vi "live data display.vi"(11 "queue":refnum<queue>) -> ()   [LabVIEW 2018]
uses:
  state.ctl
  liveData cluster.ctl
panel:
  out "STOP":bool
  out "Waveform Graph":dbl[](graph)
  in  "mode":bool
  in  "channel":u16(ring)
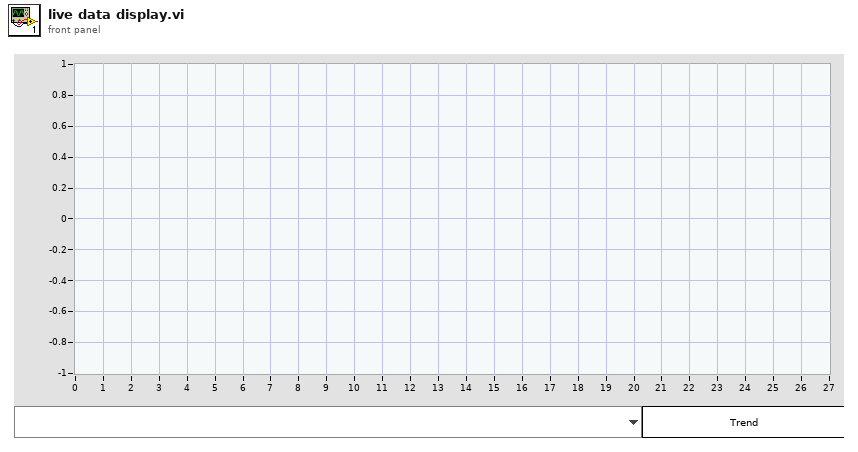
[diagram p1: front panel]
types:
  T1 = typedef "liveData cluster.ctl" = cluster{"channelSelection":i32, "length":dbl, "history":dbl[], "Trend":bool, "plotRef":refnum<vi>}
  T2 = typedef "state.ctl" = enum16{"readData", "init", "channel", "mode", "quit"}
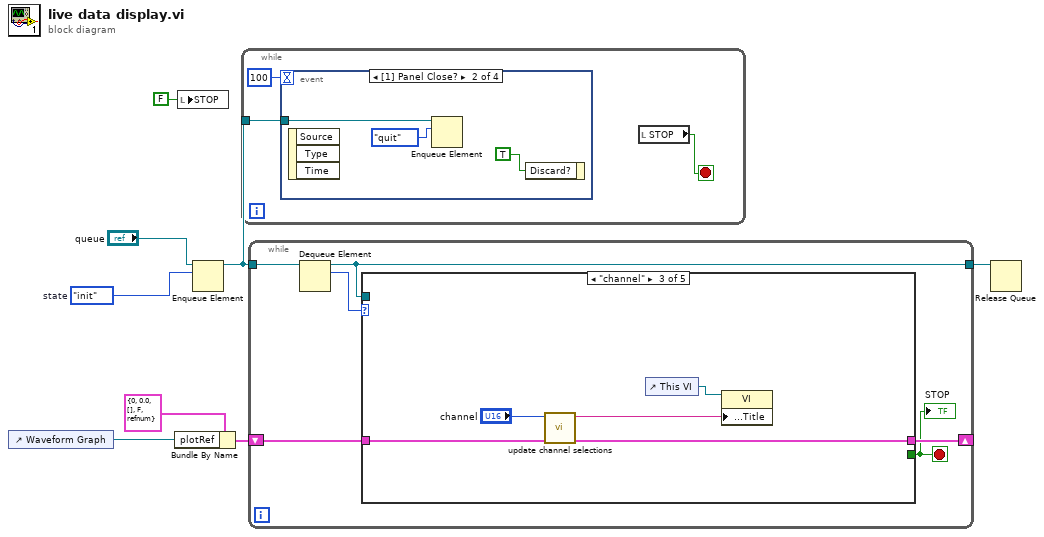
[diagram p0: block diagram]
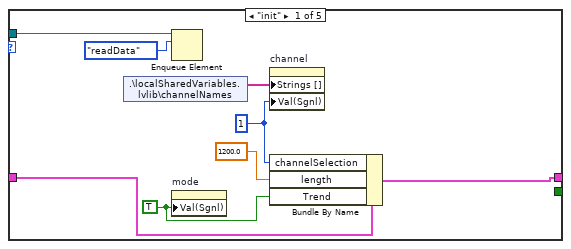
[diagram p2: hidden frame]
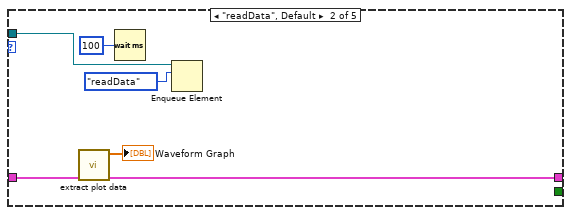
[diagram p3: hidden frame]
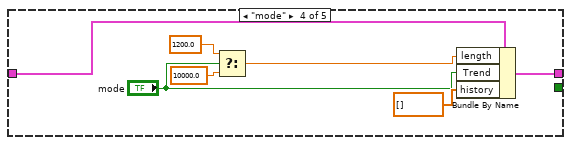
[diagram p4: hidden frame]
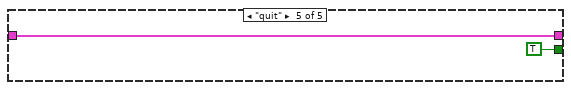
[diagram p5: hidden frame]
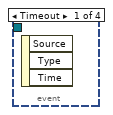
[diagram p6: hidden frame]
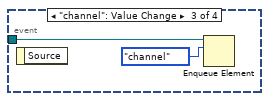
[diagram p7: hidden frame]
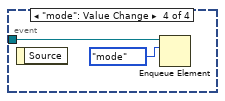
[diagram p8: hidden frame]
diagram:
  w3 = state."init"  # state
  n1 = control-ref of="Waveform Graph"() -> (w4:refnum<vi>)
  n2 = Bundle By Name(cluster=T1 {"channelSelection"=0, "length"=0.0, "history"=[], "Trend"=FALSE, "plotRef"=refnum}, "plotRef"=w4) -> (w5:T1)
  n3 = local write "STOP"(FALSE ("STOP")) -> ()
  n4 = Enqueue Element(queue="queue", element=w3) -> (queue out=w6:refnum<queue>)  [unwired: 2 in, 2 out]
  n5 = while {
    tunnel: w6 -> [w11]
    stop <- w10 stop-if-true
    n6 = event shown="[1] Panel Close?" {
      selector: _ -> [_ _ _ _]
      dyn-events: _ -> [_ _ _ _]
      timeout: 100 -> [_ _ _ _]
      tunnel: w11 -> [_ w13 w16 w18]
      event Timeout {
        n7 = event-data() -> ()  [unwired: 1 in, 3 out]
      }
      event Panel Close? {
        n8 = event-data() -> ()  [unwired: 1 in, 3 out]
        n9 = Enqueue Element(queue=w13, element=state."quit") -> ()  [unwired: 2 in, 3 out]
        n10 = event-data("Discard?"=TRUE) -> ()  [unwired: 1 in, 1 out]
      }
      event "channel": Value Change {
        n11 = event-data() -> ()  [unwired: 1 in, 1 out]
        n12 = Enqueue Element(queue=w16, element=state."channel") -> ()  [unwired: 2 in, 3 out]
      }
      event "mode": Value Change {
        n13 = event-data() -> ()  [unwired: 1 in, 1 out]
        n14 = Enqueue Element(queue=w18, element=state."mode") -> ()  [unwired: 2 in, 3 out]
      }
    }
    n15 = local read "STOP"() -> (w10:bool)
  }
  n16 = while {
    shift-right: [w22] -> _
    shift-left: w5 -> [w24]
    tunnel: w6 -> [w23]
    tunnel: [w21] -> w8
    stop <- w19 stop-if-true
    n17 = Dequeue Element(queue=w23) -> (queue out=w21:refnum<queue>, element=w20:T2)  [unwired: 2 in, 2 out]
    n18 = case shown="\"channel\"" w20 {
      tunnel: w24 -> [w32 w36 w43 w50 w51]
      tunnel: w21 -> [w30 w38 _ _ _]
      tunnel: [_ _ _ _ TRUE] -> w19
      tunnel: [w31 w35 w42 w49 w51] -> w22
      frame "init" {
        w26 = TRUE ("Trend")
        w27 = 1 ("channelSelection")
        n19 = shared-variable ".\\localSharedVariables.lvlib\\channelNames"() -> (w28:string[])  [unwired: 1 in, 1 out]
        n20 = Enqueue Element(queue=w30, element=state."readData" ("state")) -> ()  [unwired: 2 in, 3 out]
        n21 = property on="mode" class="Bool (strict)"("Val(Sgnl)"=w26) -> ()  [unwired: 2 in, 2 out]
        n22 = property on="channel" class="Ring (strict)"("Strings []"=w28, "Val(Sgnl)"=w27) -> ()  [unwired: 2 in, 2 out]
        n23 = Bundle By Name(cluster=w32, "channelSelection"=w27, "length"=1200.0, "Trend"=w26) -> (w31:T1)
      }
      frame "readData", Default {
        n24 = call "extract plot data.vi"("data in"=w36) -> ("data out"=w35:T1, "plotData"=→"Waveform Graph":dbl[])  [unwired: 9 in]
        n25 = Wait (ms)(milliseconds to wait=u32 100) -> ()  [unwired: 1 out]
        n26 = Enqueue Element(queue=w38, element=state."readData" ("state")) -> ()  [unwired: 2 in, 3 out]
      }
      frame "channel" {
        n27 = call "update channel selections.vi"("data"=w43, "channelSelection"="channel") -> ("data out"=w42:T1, "selected channel"=w40:string)  [unwired: 8 in]
        n28 = control-ref of="This VI"() -> (w39:refnum<vi>)
        n29 = property class="VI"(reference=w39, "Front Panel.Title"=w40) -> ()  [unwired: 1 in, 2 out]
      }
      frame "mode" {
        n30 = Select(t=1200.0, s="mode", f=10000.0) -> (s? t:f=w45:dbl)
        n31 = Bundle By Name(cluster=w50, "length"=w45, "Trend"="mode", "history"=dbl[] []) -> (w49:T1)
      }
      frame "quit" {
      }
    }
    "STOP" <- w19
  }
  n32 = Release Queue(queue=w8) -> ()  [unwired: 2 in, 3 out]
